vi "Write Wait Time.vi"(8 "error in (no error)":errorcluster, 10 "Wait Time in ms (0)":i32, 11 "Wait Msg in":refnum<class "Wait Msg.lvclass">) -> (0 "error out":errorcluster, 3 "Wait Msg out":refnum<class "Wait Msg.lvclass">)   [LabVIEW 2020, in "Sequencer.lvlib" / "Wait Msg.lvclass"]
doc: "Write wait time."
uses:
  Wait Msg.lvclass
  Wait Msg.lvclass/Wait Msg.ctl
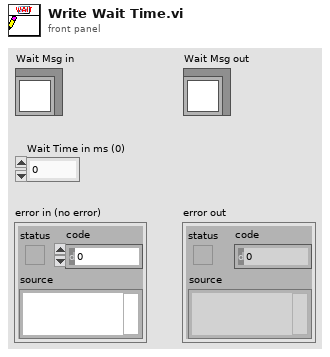
[diagram p1: front panel]
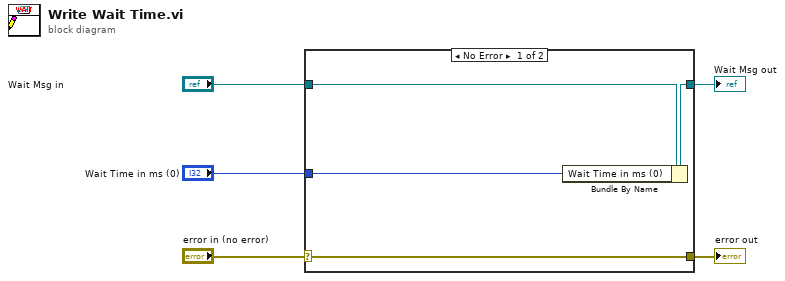
[diagram p0: block diagram]
diagram:
  n1 = case shown="No Error" "error in (no error)" {
    selector: "error in (no error)" -> [w9 w10]
    tunnel: [w9 w10] -> w4
    tunnel: [w7 w11] -> w2
    tunnel: "Wait Msg in" -> [w8 w11]
    tunnel: "Wait Time in ms (0)" -> [w6 _]
    frame No Error {
      n2 = Bundle By Name(cluster=w8, "Wait Time in ms (0)"=w6) -> (w7:refnum<class "Wait Msg.lvclass">)
    }
    frame Error {
    }
  }
  "error out" <- w4
  "Wait Msg out" <- w2
